vi "FGV_Counter Frequency divider.vi"() -> ()   [LabVIEW 2017]
doc: "This example demonstrates how to continuously generate digital pulses using a counter output."
uses:
  Controls/FV_Counter Frequency Divider.ctl
  <vilib>/DAQmx/create/channels.llb/DAQmx Create Channel (CO-Pulse Generation-Ticks).vi
  <vilib>/DAQmx/configure/timing.llb/DAQmx Timing (Implicit).vi
  <vilib>/DAQmx/configure/trigger.llb/DAQmx Start Trigger (Digital Edge).vi
  <resource>/objmgr/daqmx.rc
panel:
  in  "Edge":i32(ring)=10280 items=["Rising"=10280, "Falling"=10171]
  in  "Digital Trigger Source":tag
  in  "low ticks":u32=100
  in  "high ticks":u32=100
  in  "source of ticks":tag="OnboardClock"
  in  "FV":T1
  out "Actual Duty Cycle":dbl
  out "Actual Frequency":dbl
  in  "Output Terminal":tag="/Dev1/PFI12"
  in  "Counter":tag="Dev1/ctr0"
  # "Channel Settings"
  # "Trigger Settings"
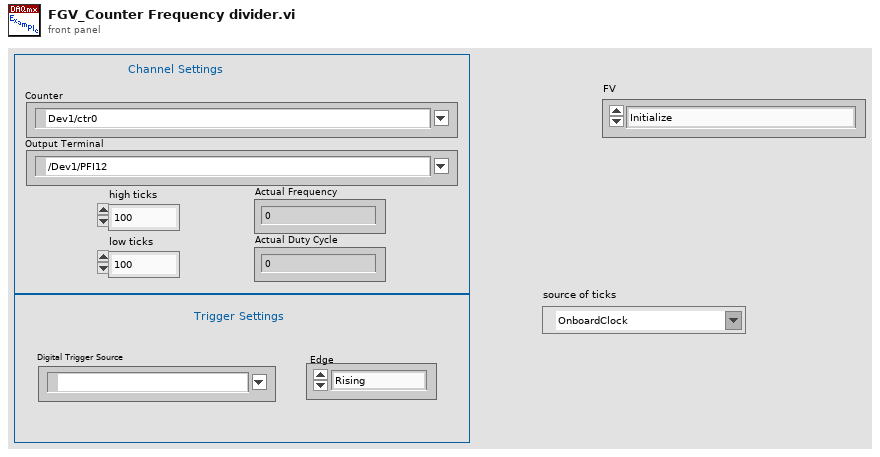
[diagram p1: front panel]
types:
  T1 = typedef "FV_Counter Frequency Divider.ctl" = enum16{"Initialize", "Channel Settings", "Timing Settings", "Trigger Settings", "Task start", "Generate Data", "Task release"}
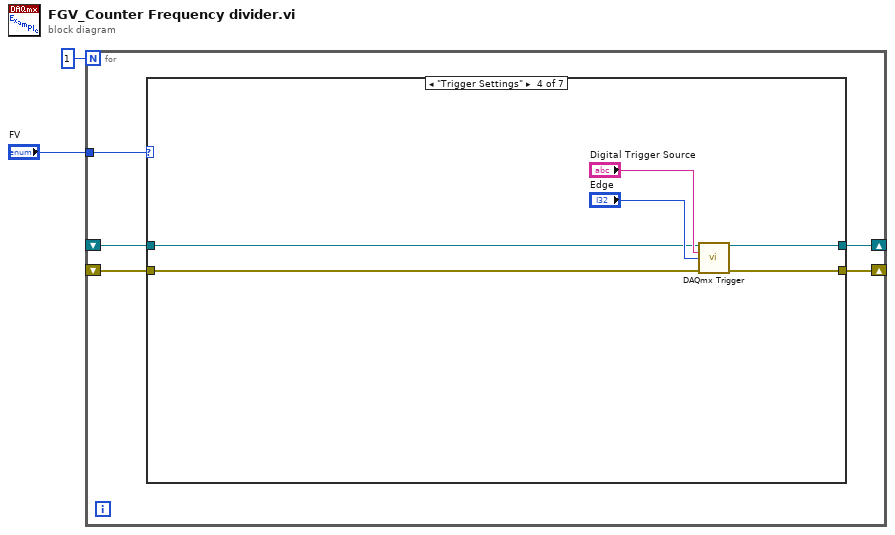
[diagram p0: block diagram]
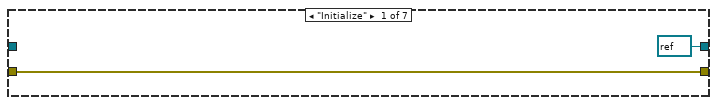
[diagram p2: hidden frame]
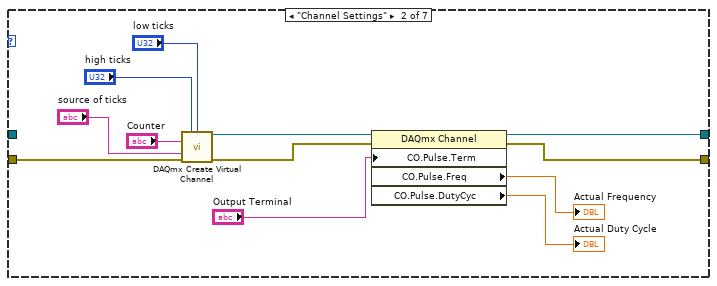
[diagram p3: hidden frame]
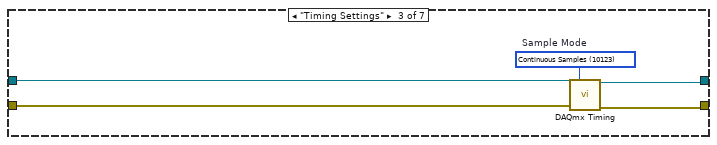
[diagram p4: hidden frame]
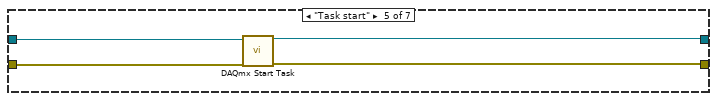
[diagram p5: hidden frame]
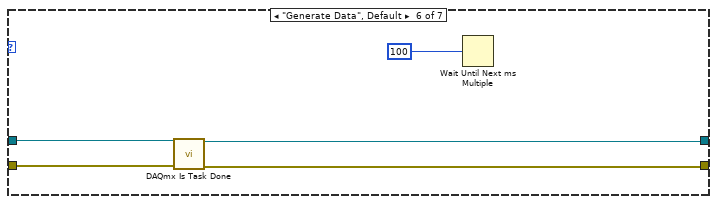
[diagram p6: hidden frame]
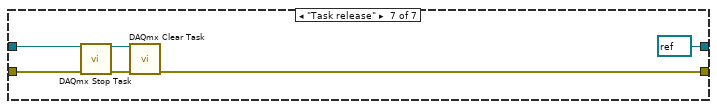
[diagram p7: hidden frame]
diagram:
  n1 = for {
    N: 1 -> [_]
    tunnel: "FV" -> [w7]
    shift-right: [w6] -> _
    shift-left: _ -> [w4]
    shift-right: [w5] -> _
    shift-left: _ -> [w3]
    n2 = case shown="\"Trigger Settings\"" w7 {
      tunnel: [refnum<k21> refnum ("task out") w17 w25 w30 w34 w38 refnum<k21> refnum ("task out")] -> w6
      tunnel: [w9 w15 w24 w29 w33 w39 w43] -> w5
      tunnel: w4 -> [_ _ w23 w28 w36 w41 w45]
      tunnel: w3 -> [w9 w19 w22 w27 w35 w40 w44]
      frame "Initialize" {
      }
      frame "Channel Settings" {
        n3 = call-poly <vilib>:"DAQmx Create Virtual Channel.vi"("high ticks"="high ticks", "low ticks"="low ticks", "counter"="Counter", "source of ticks"="source of ticks", "error in"=w19) -> ("task out"=w21:refnum<k21>, "error out"=w16:errorcluster)  [unwired: 9 in]
        n4 = property class="DAQmx Channel"(reference=w21, error in=w16, "CO.Pulse.Term"="Output Terminal") -> (reference out=w17:refnum<k21>, error out=w15:errorcluster, "CO.Pulse.Freq"=→"Actual Frequency":dbl, "CO.Pulse.DutyCyc"=→"Actual Duty Cycle":dbl)
      }
      frame "Timing Settings" {
        w26 = 10123 items=["Finite Samples"=10178, "Continuous Samples"=10123, "Hardware Timed Single Point"=12522]  # Sample Mode
        n5 = call-poly <vilib>:"DAQmx Timing.vi"("task/channels in"=w23, "sample mode"=w26, "error in"=w22) -> ("task out"=w25:refnum<k21>, "error out"=w24:errorcluster)  [unwired: 11 in]
      }
      frame "Trigger Settings" {
        n6 = call-poly <vilib>:"DAQmx Trigger.vi"("task/channels in"=w28, "source"="Digital Trigger Source", "edge"="Edge", "error in"=w27) -> ("task out"=w30:refnum<k21>, "error out"=w29:errorcluster)  [unwired: 10 in]
      }
      frame "Task start" {
        n7 = call <vilib>:"DAQmx Start Task.vi"("task/channels in"=w36, "error in"=w35) -> ("task out"=w34:refnum<k21>, "error out"=w33:errorcluster)  [unwired: 12 in]
      }
      frame "Generate Data", Default {
        n8 = call <vilib>:"DAQmx Is Task Done.vi"("task/channels in"=w41, "error in"=w40) -> ("task out"=w38:refnum<k21>, "error out"=w39:errorcluster)  [unwired: 11 in, 1 out]
        n9 = Wait Until Next ms Multiple(millisecond multiple=u32 100) -> ()  [unwired: 1 out]
      }
      frame "Task release" {
        n10 = call <vilib>:"DAQmx Stop Task.vi"("task/channels in"=w45, "error in"=w44) -> ("task out"=w46:refnum<k21>, "error out"=w47:errorcluster)  [unwired: 12 in]
        n11 = call <vilib>:"DAQmx Clear Task.vi"("task in"=w46, "error in"=w47) -> ("error out"=w43:errorcluster)  [unwired: 13 in]
      }
    }
  }
